vi "TLPM_PowerMeter_Sample.vi"() -> ()   [LabVIEW 2017]
panel:
  out "Active":bool
  in  "stop":bool
  out "Power Value":dbl caption="Optical Power [W]" format="%#_4p"
  # "TLPM"
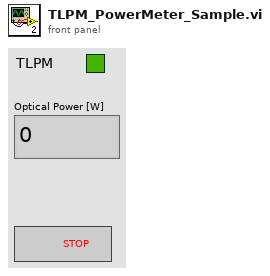
[diagram p1: front panel]
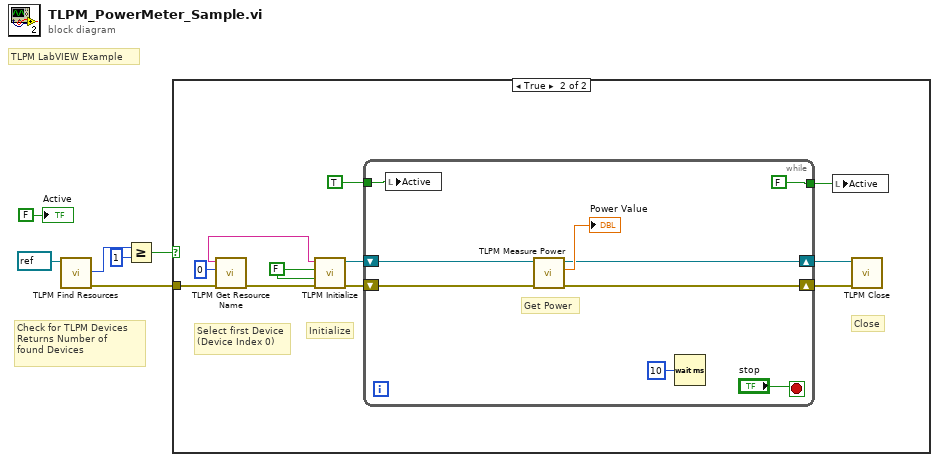
[diagram p0: block diagram]
diagram:
  # "TLPM LabVIEW Example"
  # "Check for TLPM Devices\nReturns Number of\nfound Devices"
  n1 = call <instrlib>:"TLPM Find Resources.vi"("instrument handle"=refnum<visa-resource-name> refnum) -> ("error out"=w5:errorcluster, "Resource Count"=w3:u32)  [unwired: 8 in, 1 out]
  n2 = Greater Or Equal?(x=w3, y=u32 1) -> (x >= y?=w4:bool)
  n3 = case shown="True" w4 {
    tunnel: w5 -> [_ w13]
    frame False {
    }
    frame True {
      w11 = FALSE ("ID Query (Do Query)")
      # "Close"
      # "Initialize"
      # "Select first Device\n(Device Index 0)"
      n4 = call <instrlib>:"TLPM Get Resource Name.vi"("error in (no error)"=w13, "Index (0)"=u32 0 ("Device Index")) -> ("error out"=w16:errorcluster, "Resource Name"=w14:string)  [unwired: 7 in, 1 out]
      n5 = call <instrlib>:"TLPM Initialize.vi"("error in (no error)"=w16, "Reset Device (Reset Device)"=w11, "ID Query (Do Query)"=w11, "resource name"=w14) -> ("error out"=w9:errorcluster, "instrument handle out"=w10:refnum<visa-resource-name>)  [unwired: 6 in]
      n6 = while {
        shift-right: [w19] -> w17
        shift-left: w10 -> [w25]
        shift-right: [w18] -> w15
        shift-left: w9 -> [w24]
        tunnel: [FALSE ("Active")] -> w8
        tunnel: TRUE ("Active") -> [w20]
        stop <- "stop" stop-if-true
        # "Get Power"
        n7 = local write "Active"(w20) -> ()
        n8 = call <instrlib>:"TLPM Measure Power.vi"("error in (no error)"=w24, "instrument handle"=w25) -> ("error out"=w18:errorcluster, "Power"=→"Power Value":dbl, "instrument handle out"=w19:refnum<visa-resource-name>)  [unwired: 7 in]
        n9 = Wait (ms)(milliseconds to wait=u32 10) -> ()  [unwired: 1 out]
      }
      n10 = local write "Active"(w8) -> ()
      n11 = call <instrlib>:"TLPM Close.vi"("error in (no error)"=w15, "instrument handle"=w17) -> ()  [unwired: 9 in, 1 out]
    }
  }
  "Active" <- FALSE ("Active")
